vi "KepcoDCPwr Clear All Lists.vi"(0 "VISA Session":refnum<visa-resource-name>, 5 "Model In":string, 7 "channel name (\"\")":string="\"\"", 11 "error in (no error)":errorcluster {"code" format="%.0x"}) -> (4 "VISA Session Out":refnum<visa-resource-name>, 6 "Model Out":string, 8 "channel name out (\"\")":string="\"\"" caption="channel name Out (\"\")", 15 "error out":errorcluster {"code" format="%.0x"})   [LabVIEW 2020]
doc: "This VI clear all list stored in instrument.\n\nNote:\n\n1) This VI does not change operational status of Power supply\n2. This Vi should be used before loading a list to insure the list is empty. \nThe initializize VI does not clear lists."
uses:
  Match Regular Expression.xnode
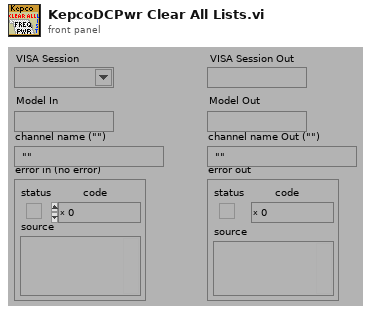
[diagram p1: front panel]
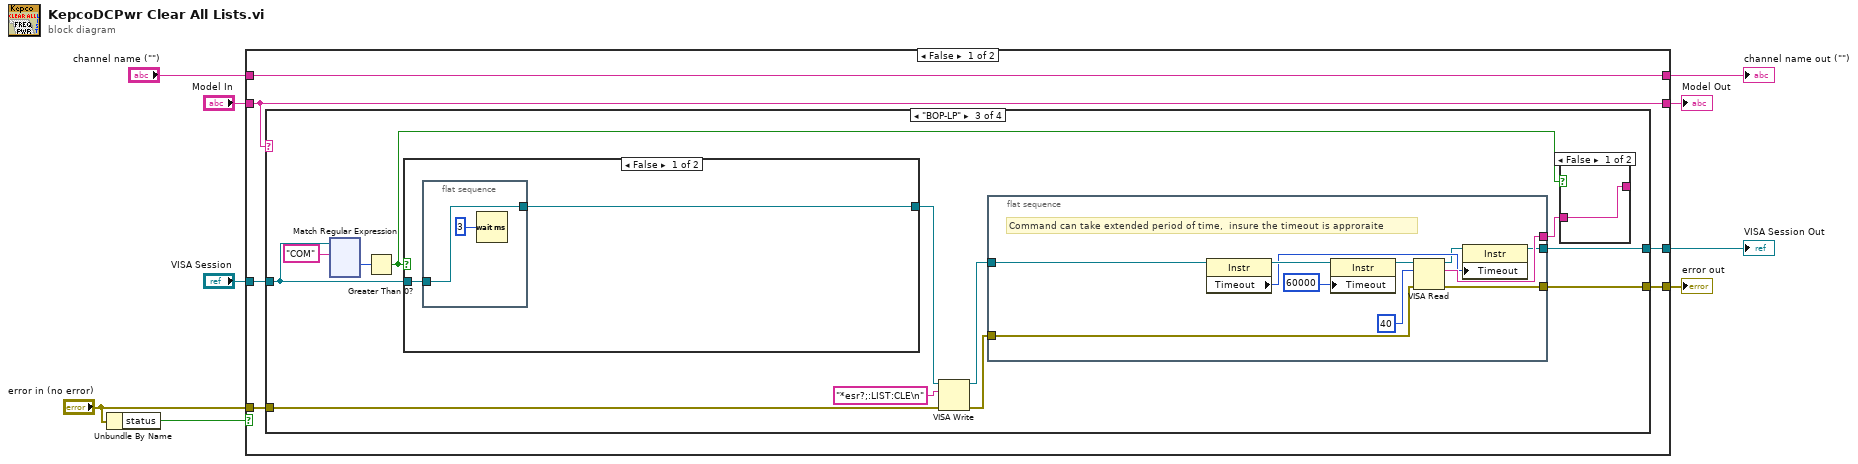
[diagram p0: block diagram]
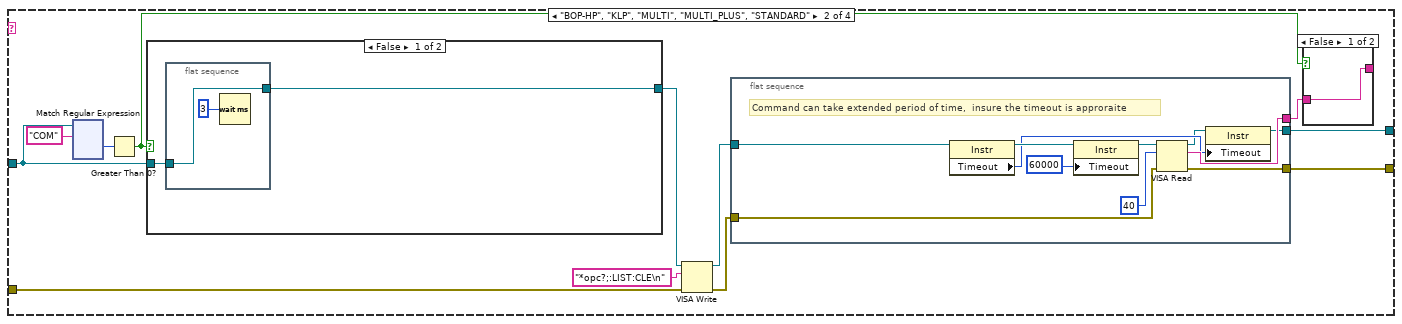
[diagram p3: hidden frame]
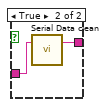
[diagram p4: hidden frame]
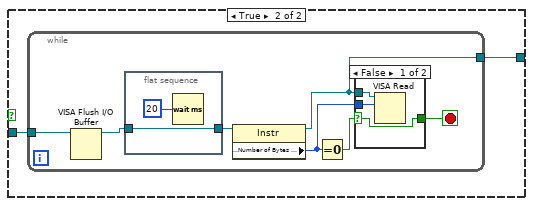
[diagram p5: hidden frame]
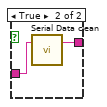
[diagram p7: hidden frame]
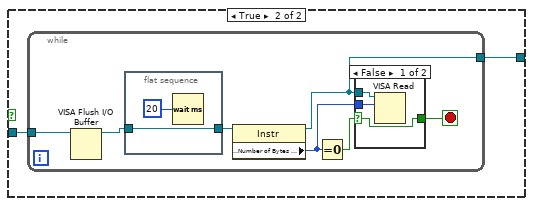
[diagram p8: hidden frame]
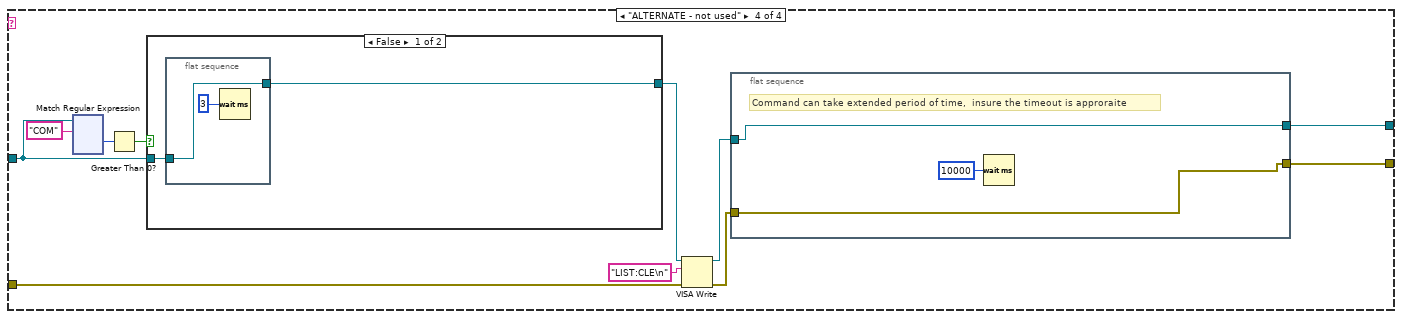
[diagram p10: hidden frame]
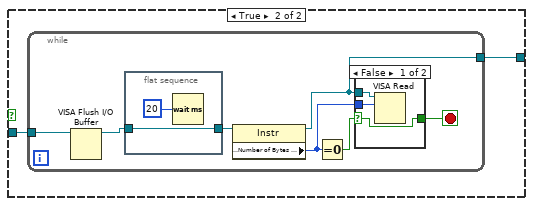
[diagram p11: hidden frame]
diagram:
  n1 = Unbundle By Name("error in (no error)") -> ("status"=w8:bool)
  n2 = case shown="False" w8 {
    tunnel: [w11 w477] -> w9
    tunnel: "error in (no error)" -> [w10 w477]
    tunnel: [w12 w476] -> w1
    tunnel: "VISA Session" -> [w13 w476]
    tunnel: [w14 w475] -> w2
    tunnel: "Model In" -> [w14 w475]
    tunnel: [w15 w474] -> w3
    tunnel: "channel name (\"\")" -> [w15 w474]
    frame False {
      n3 = case shown="\"BOP-LP\"" w14 {
        tunnel: w10 -> [w17 w29 w185 w340]
        tunnel: [w17 w20 w176 w332] -> w11
        tunnel: w13 -> [w16 w25 w181 w336]
        tunnel: [w16 w18 w174 w330] -> w12
        frame "", Default {
        }
        frame "BOP-HP", "KLP", "MULTI", "MULTI_PLUS", "STANDARD" {
          n4 = xnode "Match Regular Expression"("input string"=w25, "regular expression"="COM") -> ("offset past match"=w26:i32)  [unwired: 2 in, 6 out]
          n5 = Greater Than 0?(x=w26) -> (x > 0?=w22:bool)
          n6 = case shown="False" w22 {
            tunnel: [w45 w49] -> w24
            tunnel: w25 -> [w44 w48]
            frame False {
              n7 = flat-sequence {
                tunnel: w44 -> [w47]
                tunnel: [w47] -> w45
                frame #0 {
                  n8 = Wait (ms)(milliseconds to wait=u32 3 ("byte count (0)")) -> ()  [unwired: 1 out]
                }
              }
            }
            frame True {
              n9 = while {
                tunnel: w48 -> [w52]
                tunnel: [w54] -> w49
                stop <- w55 stop-if-true
                n10 = VISA Flush I/O Buffer(VISA resource name=w52) -> (VISA resource name out=w51:refnum<visa-resource-name>)  [unwired: 2 in, 1 out]
                n11 = flat-sequence {
                  tunnel: w51 -> [w57]
                  tunnel: [w57] -> w50
                  frame #0 {
                    n12 = Wait (ms)(milliseconds to wait=u32 20) -> ()  [unwired: 1 out]
                  }
                }
                n13 = property class="Instr"(reference=w50) -> (reference out=w54:refnum<visa-resource-name>, "Serial Settings:Number of Bytes at Serial Port"=w53:u32)  [unwired: 1 in, 1 out]
                n14 = Equal To 0?(x=w53) -> (x = 0?=w56:bool)
                n15 = case shown="False" w56 {
                  selector: w56 -> [w61 w62]
                  tunnel: [w61 w62] -> w55
                  tunnel: w54 -> [w60 _]
                  tunnel: w53 -> [w59 _]
                  frame False {
                    n16 = VISA Read(VISA resource name=w60, byte count=w59) -> ()  [unwired: 1 in, 4 out]
                  }
                  frame True {
                  }
                }
              }
            }
          }
          n17 = VISA Write(VISA resource name=w24, write buffer="*opc?;:LIST:CLE\n", error in (no error)=w29) -> (VISA resource name out=w19:refnum<visa-resource-name>, error out=w21:errorcluster)  [unwired: 1 out]
          n18 = flat-sequence {
            tunnel: [w40] -> w23
            tunnel: w21 -> [w39]
            tunnel: [w38] -> w20
            tunnel: w19 -> [w37]
            tunnel: [w32] -> w18
            frame #0 {
              # "Command can take extended period of time,  insure the timeout is approraite"
              n19 = property class="Instr"(reference=w37) -> (reference out=w36:refnum<visa-resource-name>, "Timeout"=w34:u32)  [unwired: 1 in, 1 out]
              n20 = property class="Instr"(reference=w36, "Timeout"=u32 60000 ("General Settings:Timeout Value")) -> (reference out=w31:refnum<visa-resource-name>)  [unwired: 1 in, 1 out]
              n21 = VISA Read(VISA resource name=w31, byte count=u32 40, error in (no error)=w39) -> (VISA resource name out=w33:refnum<visa-resource-name>, read buffer=w40:string, error out=w38:errorcluster)  [unwired: 1 out]
              n22 = property class="Instr"(reference=w33, "Timeout"=w34) -> (reference out=w32:refnum<visa-resource-name>)  [unwired: 1 in, 1 out]
            }
          }
          n23 = case shown="False" w22 {
            tunnel: w23 -> [w41 w42]
            tunnel: [w41 w43] -> _
            frame False {
            }
            frame True {
              n24 = call "Serial Data clean.vi"("string"=w42) -> ("Stripped of Xon Xoff"=w43:string)  [unwired: 2 in]
            }
          }
        }
        frame "BOP-LP" {
          n25 = xnode "Match Regular Expression"("input string"=w181, "regular expression"="COM") -> ("offset past match"=w182:i32)  [unwired: 2 in, 6 out]
          n26 = Greater Than 0?(x=w182) -> (x > 0?=w178:bool)
          n27 = case shown="False" w178 {
            tunnel: [w201 w205] -> w180
            tunnel: w181 -> [w200 w204]
            frame False {
              n28 = flat-sequence {
                tunnel: w200 -> [w203]
                tunnel: [w203] -> w201
                frame #0 {
                  n29 = Wait (ms)(milliseconds to wait=u32 3 ("byte count (0)")) -> ()  [unwired: 1 out]
                }
              }
            }
            frame True {
              n30 = while {
                tunnel: w204 -> [w208]
                tunnel: [w210] -> w205
                stop <- w211 stop-if-true
                n31 = VISA Flush I/O Buffer(VISA resource name=w208) -> (VISA resource name out=w207:refnum<visa-resource-name>)  [unwired: 2 in, 1 out]
                n32 = flat-sequence {
                  tunnel: w207 -> [w213]
                  tunnel: [w213] -> w206
                  frame #0 {
                    n33 = Wait (ms)(milliseconds to wait=u32 20) -> ()  [unwired: 1 out]
                  }
                }
                n34 = property class="Instr"(reference=w206) -> (reference out=w210:refnum<visa-resource-name>, "Serial Settings:Number of Bytes at Serial Port"=w209:u32)  [unwired: 1 in, 1 out]
                n35 = Equal To 0?(x=w209) -> (x = 0?=w212:bool)
                n36 = case shown="False" w212 {
                  selector: w212 -> [w217 w218]
                  tunnel: [w217 w218] -> w211
                  tunnel: w210 -> [w216 _]
                  tunnel: w209 -> [w215 _]
                  frame False {
                    n37 = VISA Read(VISA resource name=w216, byte count=w215) -> ()  [unwired: 1 in, 4 out]
                  }
                  frame True {
                  }
                }
              }
            }
          }
          n38 = VISA Write(VISA resource name=w180, write buffer="*esr?;:LIST:CLE\n", error in (no error)=w185) -> (VISA resource name out=w175:refnum<visa-resource-name>, error out=w177:errorcluster)  [unwired: 1 out]
          n39 = flat-sequence {
            tunnel: [w196] -> w179
            tunnel: w177 -> [w195]
            tunnel: [w194] -> w176
            tunnel: w175 -> [w193]
            tunnel: [w188] -> w174
            frame #0 {
              # "Command can take extended period of time,  insure the timeout is approraite"
              n40 = property class="Instr"(reference=w193) -> (reference out=w192:refnum<visa-resource-name>, "Timeout"=w190:u32)  [unwired: 1 in, 1 out]
              n41 = property class="Instr"(reference=w192, "Timeout"=u32 60000 ("General Settings:Timeout Value")) -> (reference out=w187:refnum<visa-resource-name>)  [unwired: 1 in, 1 out]
              n42 = VISA Read(VISA resource name=w187, byte count=u32 40, error in (no error)=w195) -> (VISA resource name out=w189:refnum<visa-resource-name>, read buffer=w196:string, error out=w194:errorcluster)  [unwired: 1 out]
              n43 = property class="Instr"(reference=w189, "Timeout"=w190) -> (reference out=w188:refnum<visa-resource-name>)  [unwired: 1 in, 1 out]
            }
          }
          n44 = case shown="False" w178 {
            tunnel: w179 -> [w197 w198]
            tunnel: [w197 w199] -> _
            frame False {
            }
            frame True {
              n45 = call "Serial Data clean.vi"("string"=w198) -> ("Stripped of Xon Xoff"=w199:string)  [unwired: 2 in]
            }
          }
        }
        frame "ALTERNATE - not used" {
          n46 = xnode "Match Regular Expression"("input string"=w336, "regular expression"="COM") -> ("offset past match"=w337:i32)  [unwired: 2 in, 6 out]
          n47 = Greater Than 0?(x=w337) -> (x > 0?=w334:bool)
          n48 = case shown="False" w334 {
            tunnel: [w345 w349] -> w335
            tunnel: w336 -> [w344 w348]
            frame False {
              n49 = flat-sequence {
                tunnel: w344 -> [w347]
                tunnel: [w347] -> w345
                frame #0 {
                  n50 = Wait (ms)(milliseconds to wait=u32 3 ("byte count (0)")) -> ()  [unwired: 1 out]
                }
              }
            }
            frame True {
              n51 = while {
                tunnel: w348 -> [w352]
                tunnel: [w354] -> w349
                stop <- w355 stop-if-true
                n52 = VISA Flush I/O Buffer(VISA resource name=w352) -> (VISA resource name out=w351:refnum<visa-resource-name>)  [unwired: 2 in, 1 out]
                n53 = flat-sequence {
                  tunnel: w351 -> [w357]
                  tunnel: [w357] -> w350
                  frame #0 {
                    n54 = Wait (ms)(milliseconds to wait=u32 20) -> ()  [unwired: 1 out]
                  }
                }
                n55 = property class="Instr"(reference=w350) -> (reference out=w354:refnum<visa-resource-name>, "Serial Settings:Number of Bytes at Serial Port"=w353:u32)  [unwired: 1 in, 1 out]
                n56 = Equal To 0?(x=w353) -> (x = 0?=w356:bool)
                n57 = case shown="False" w356 {
                  selector: w356 -> [w361 w362]
                  tunnel: [w361 w362] -> w355
                  tunnel: w354 -> [w360 _]
                  tunnel: w353 -> [w359 _]
                  frame False {
                    n58 = VISA Read(VISA resource name=w360, byte count=w359) -> ()  [unwired: 1 in, 4 out]
                  }
                  frame True {
                  }
                }
              }
            }
          }
          n59 = VISA Write(VISA resource name=w335, write buffer="LIST:CLE\n", error in (no error)=w340) -> (VISA resource name out=w331:refnum<visa-resource-name>, error out=w333:errorcluster)  [unwired: 1 out]
          n60 = flat-sequence {
            tunnel: w333 -> [w342]
            tunnel: [w342] -> w332
            tunnel: w331 -> [w343]
            tunnel: [w343] -> w330
            frame #0 {
              # "Command can take extended period of time,  insure the timeout is approraite"
              n61 = Wait (ms)(milliseconds to wait=u32 10000) -> ()  [unwired: 1 out]
            }
          }
        }
      }
    }
    frame True {
    }
  }
  "error out" <- w9
  "channel name out (\"\")" <- w3
  "Model Out" <- w2
  "VISA Session Out" <- w1
